vi "UDP Data Link - Driver Utilities - TimeStamp SequenceNumber FGV.vi"(8 "error in (no error)":errorcluster, 9 "Enum":enum16{"Get", "Set"}(ring), 10 "Sequence Number In":u32, 11 "Timestamp In":dbl) -> (0 "error out":errorcluster, 2 "Sequence Number Out":u32, 3 "Timestamp Out":dbl)   [LabVIEW 2012, in "UDP Data Link Engine.lvlib"]
doc: "This is a FGV for the Sequence Number in the header of the packets to/from Simulation Machine. The UDP Tx loop should update this FGV with the most recent Sequence Number sent, and the UDP Rx loop should check the sequence number obtained in its header with the value in this FGV to make sure that there is no Sequence Number mismatch."
uses:
  UDP Data Link Engine.lvlib
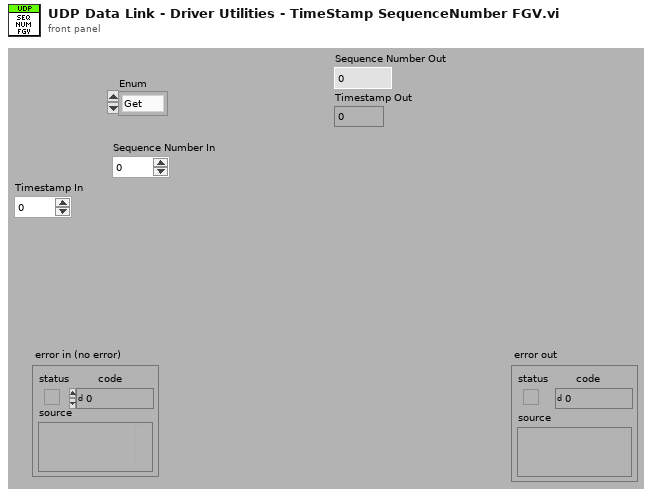
[diagram p1: front panel]
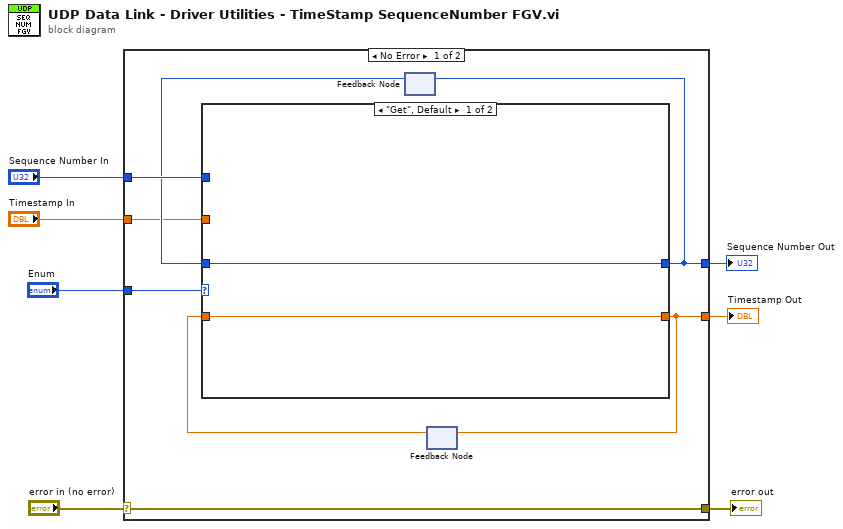
[diagram p0: block diagram]
diagram:
  n1 = case shown="No Error" "error in (no error)" {
    selector: "error in (no error)" -> [w11 w22]
    tunnel: [w11 w22] -> w6
    tunnel: "Enum" -> [w15 _]
    tunnel: "Sequence Number In" -> [w14 w21]
    tunnel: [w13 w21] -> w3
    tunnel: "Timestamp In" -> [w10 w20]
    tunnel: [w8 w20] -> w1
    frame No Error {
      n2 = feedback #1() -> (w12:u32)  [unwired: 1 in]
      n3 = feedback #2() -> (w9:dbl)  [unwired: 1 in]
      n4 = case shown="\"Get\", Default" w15 {
        tunnel: w14 -> [_ w19]
        tunnel: [w17 w19] -> w13
        tunnel: w12 -> [w17 _]
        tunnel: w10 -> [_ w18]
        tunnel: [w16 w18] -> w8
        tunnel: w9 -> [w16 _]
        frame "Get", Default {
        }
        frame "Set" {
        }
      }
      n5 = feedback-in #1(w13) -> ()
      n6 = feedback-in #2(w8) -> ()
    }
    frame Error {
    }
  }
  "error out" <- w6
  "Sequence Number Out" <- w3
  "Timestamp Out" <- w1
